vi "Step_Delay_Tommaso.vi"() -> ()   [LabVIEW 2015]
uses:
  <vilib>/DAQmx/write.llb/DAQmx Write (Analog DBL 1Chan 1Samp).vi
  <vilib>/DAQmx/miscellaneous.llb/DAQmx Fill In Error Info.vi
  <vilib>/DAQmx/create/channels.llb/DAQmx Create Channel (AO-Voltage-Basic).vi
  <vilib>/Analysis/1siggen.llb/Ramp Pattern by Delta.vi
  subvi/Newport ESP301/Newport ESP301.lvlib
  <vilib>/Analysis/NI_AALBase.lvlib
panel:
  in  "Dwell_positions":string[][](table)=[["-500", "3000"], ["-100", "3000"], ["0", "5000"], ["100", "5000"], ["500", "5000"], ["750", "10000"], ["1000", "10000"], ["", ""]]
  in  "Enable2":bool caption="Enable?"
  in  "Wait time [ms]":u32=1000 caption="Values <50 \nwon't work"
  out "StepSize [mm]":dbl=0.14989622900000002
  in  "stop 2":bool
  in  "StepSize [fs]":i32=1000
  in  "Enable?":bool
  out "a":waveform(dbl)(graph)={"t0"=timestamp(3629703941.150015 s since 1904-01-01), "dt"=1.0, "Y"=[-1.00695]}
  out "Waveform Chart":dbl(graph)=5.25341140860948
  out "x*y":dbl=0.9998993703837595
  in  "physical channels":tag="Dev3/ao1"
  out "DAC error":errorcluster
  out "ESP error":errorcluster
  out "run?":bool
  in  "set_vel":bool
  in  "velocity [fs/s]":dbl=333.564095198152
  in  "vel_mm":dbl=0.05 caption="velocity [mm/s]"
  out "meas. velocity":dbl
  in  "stop":bool
  out "output voltage":dbl=0.9998993703837595
  in  "start":bool
  in  "go2p1":bool
  out "position [mm]":dbl=-1.00695
  in  "p2 [mm]":dbl=-0.707153771
  in  "p1 [mm]":dbl=-1.006946229
  in  "interpolate output":bool
  in  "Delta2 [fs]":dbl=999.9999999999999
  in  "Delta1 [fs]":dbl=-999.9999999999999
  in  "Reference [mm]":dbl=-0.85705
  in  "Axis (1)":i32=3 min=1 max=3
  in  "Serial Link (RS232)":enum16{"RS232", "USB"}(ring)
  in  "VISA resource name":refnum<visa-resource-name>="COM9"
  in  "main_close":bool
  # "Interface panel"
  # "Velocity panel"
  # "Positions panel"
  # "Equally spaced steps panel"
  # "Controls panel"
  # "User-defined steps panel"
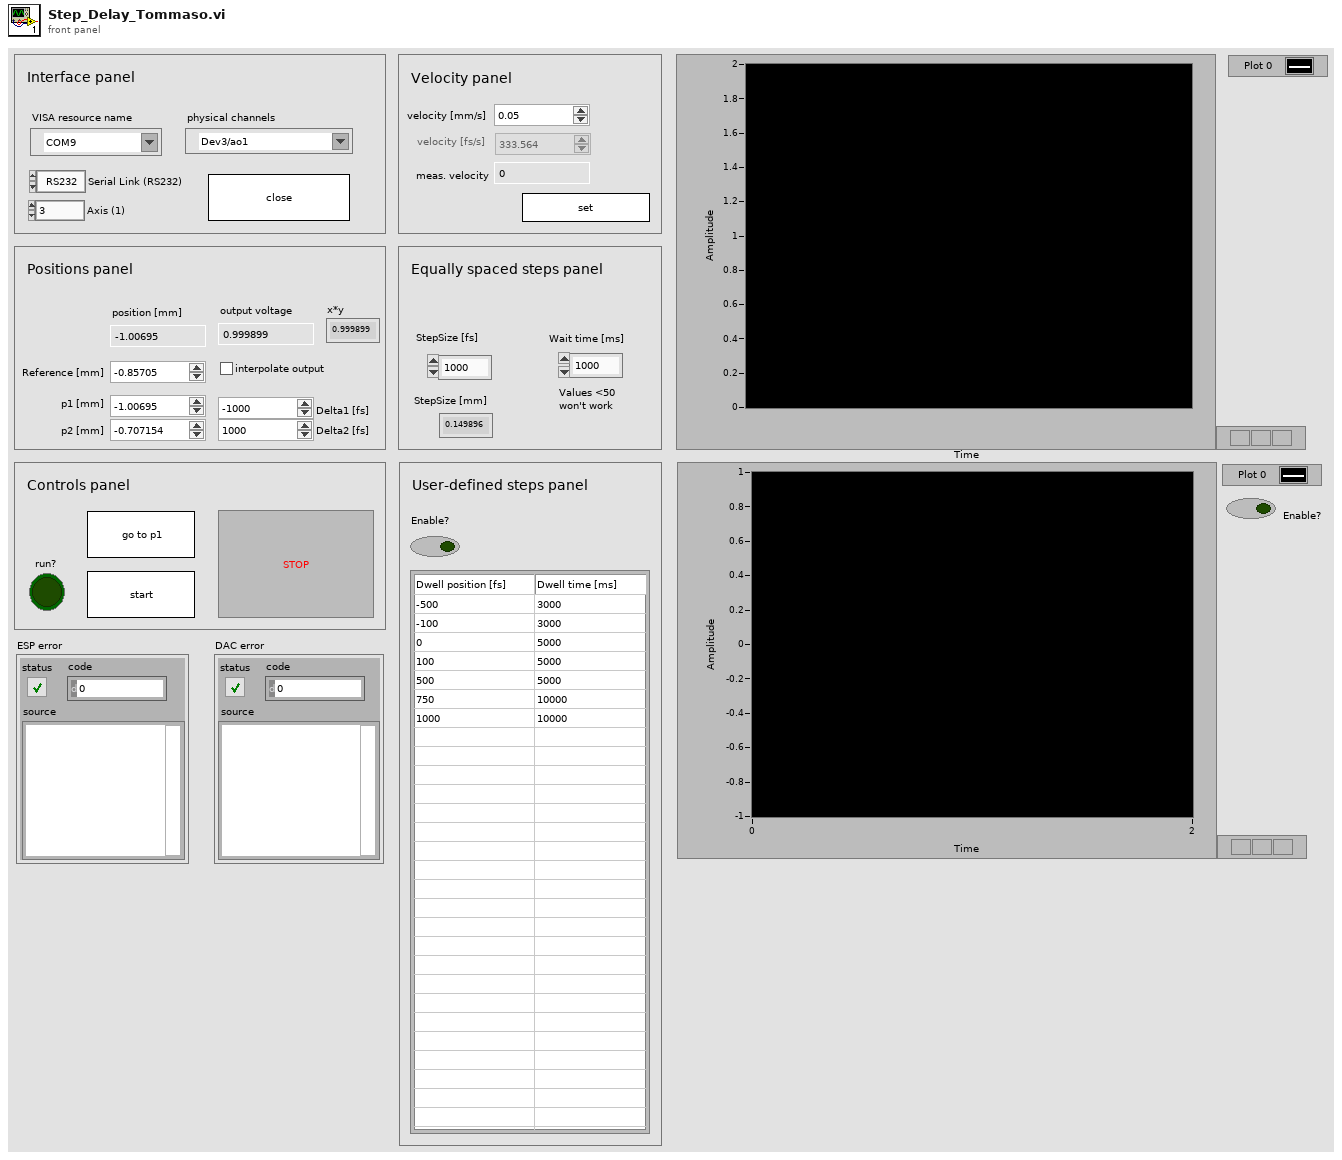
[diagram p1: front panel]
types:
  T1 = cluster{"dev1_data":refnum<queue>, "dev2_data":refnum<queue>}
  T2 = cluster{"dev1_cmd":refnum<queue>, "dev2_cmd":refnum<queue>}
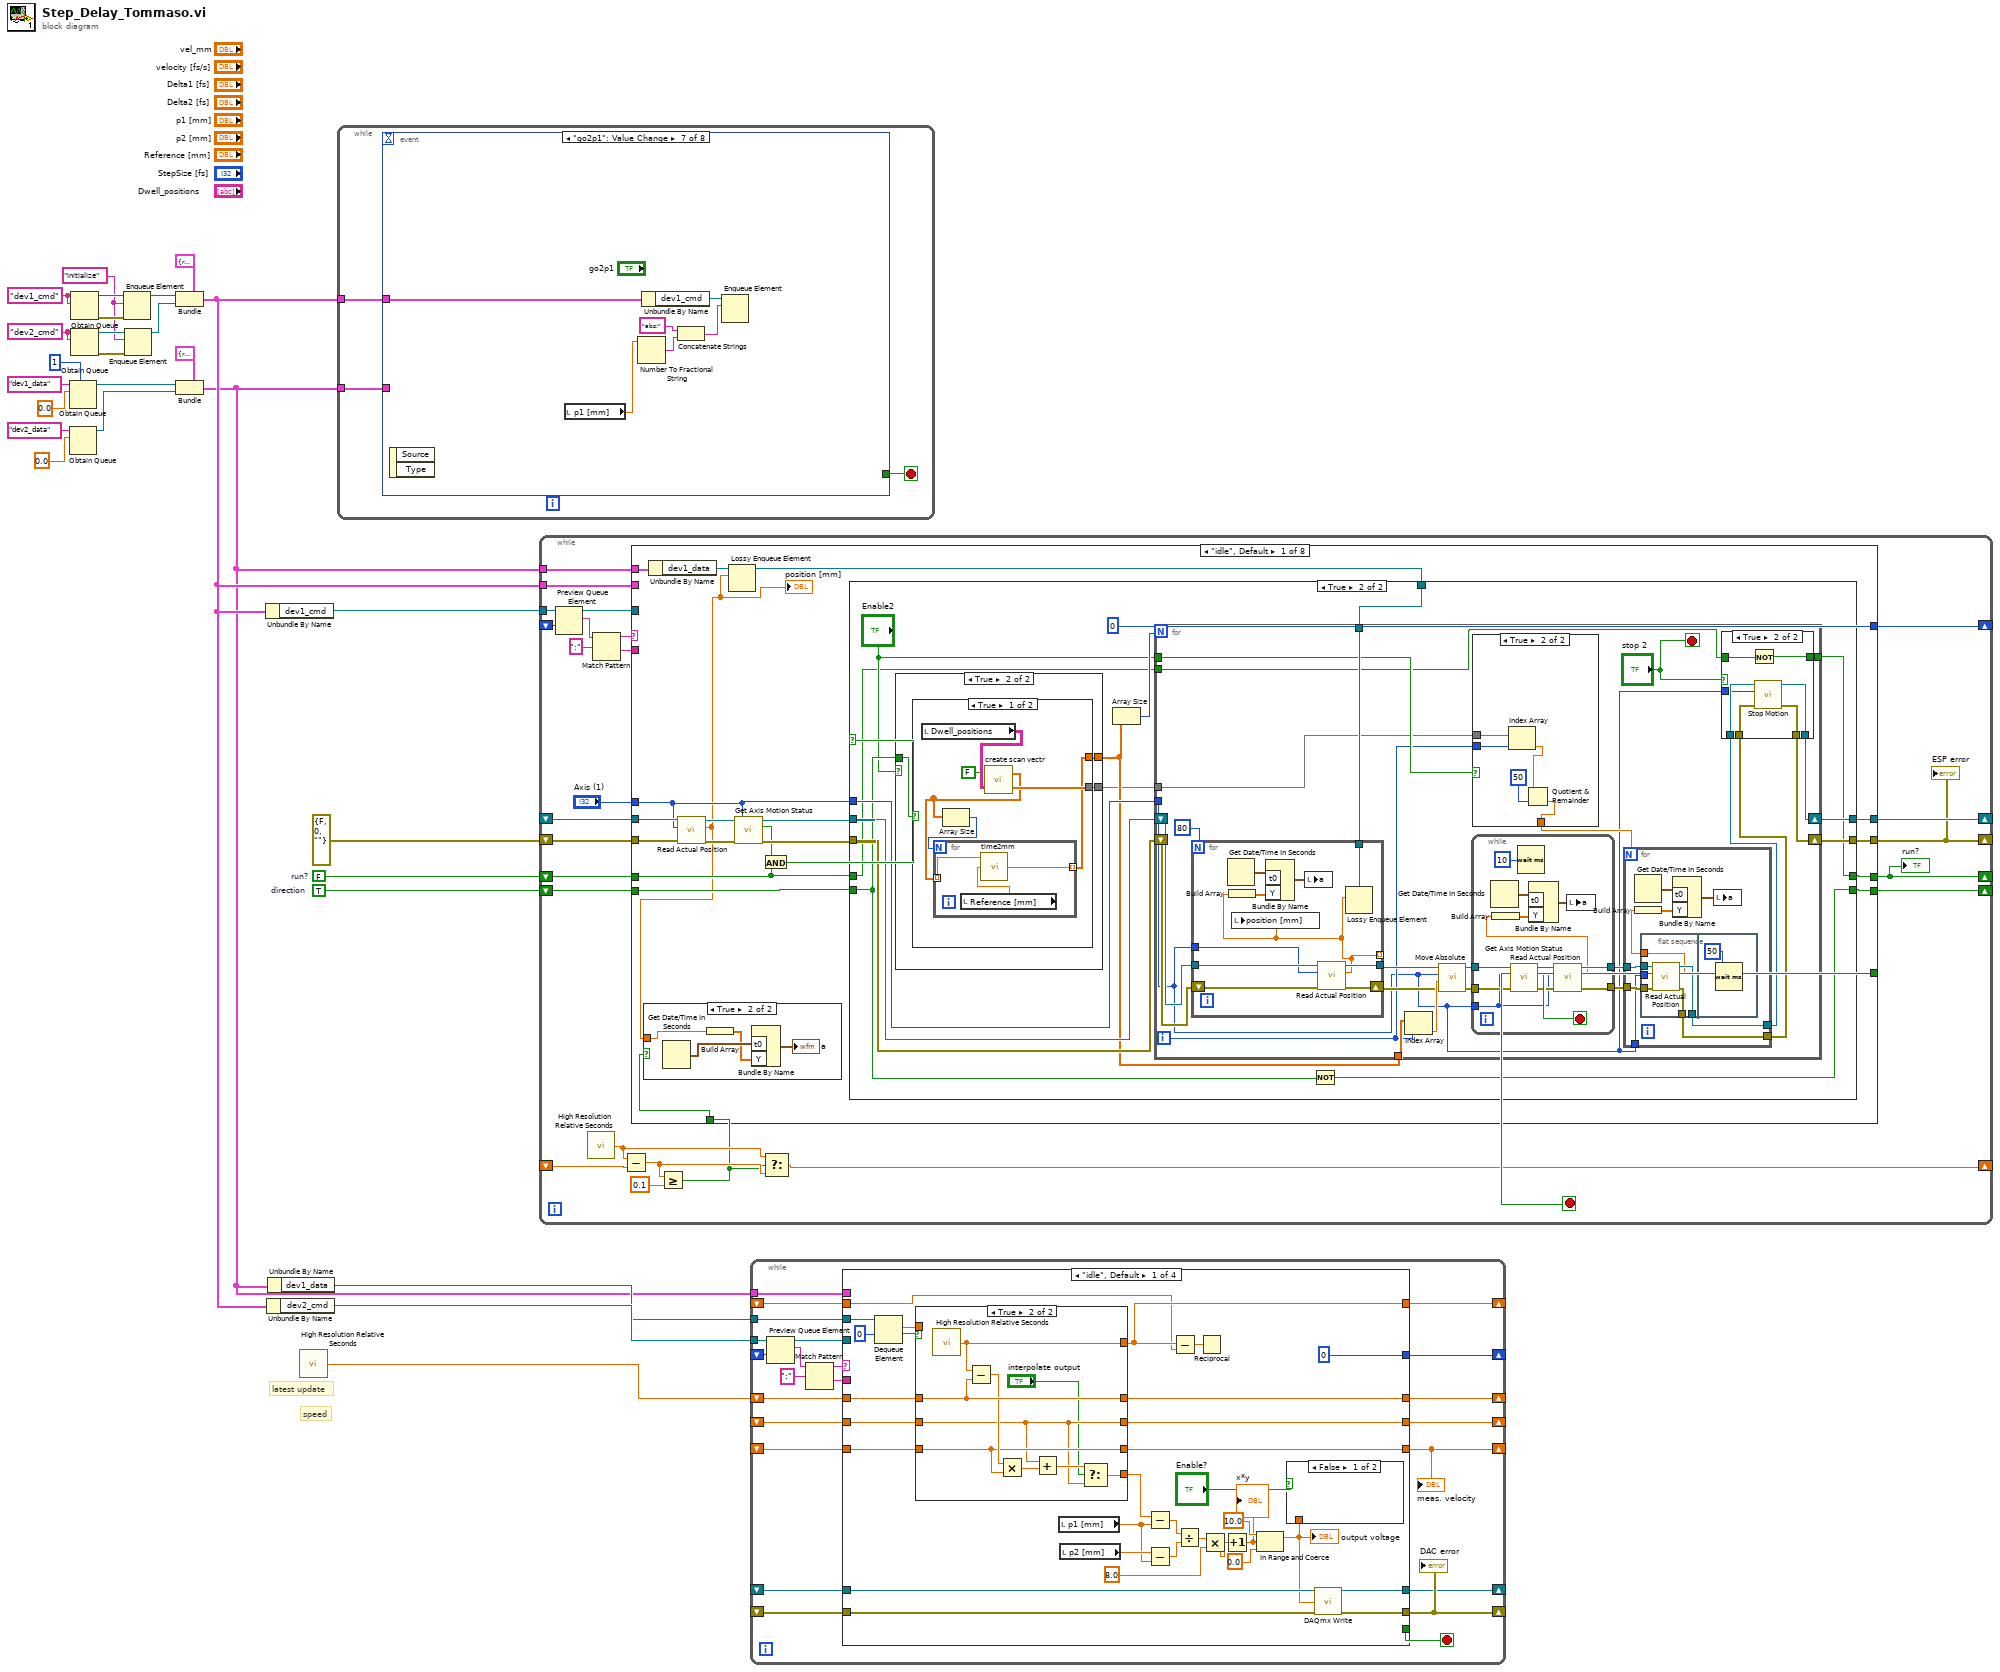
[diagram p0: block diagram]
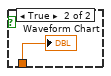
[diagram p2: hidden frame]
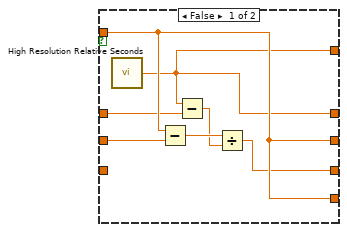
[diagram p3: hidden frame]
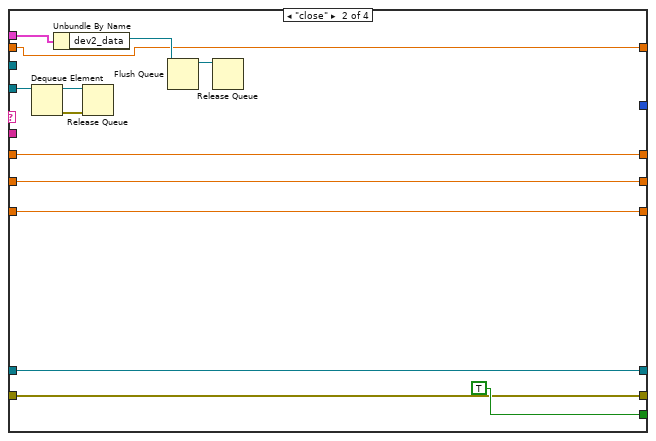
[diagram p4: hidden frame]
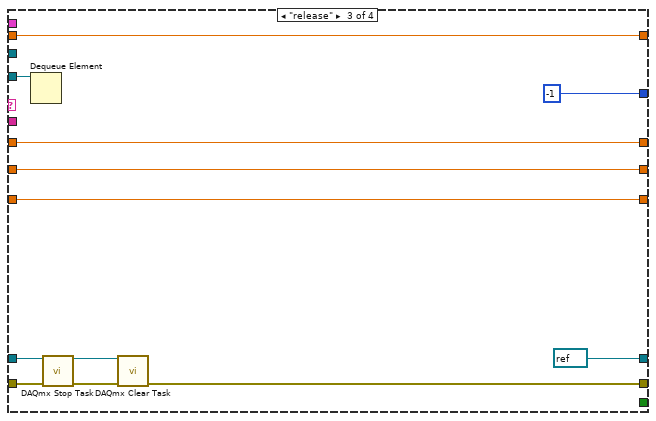
[diagram p5: hidden frame]
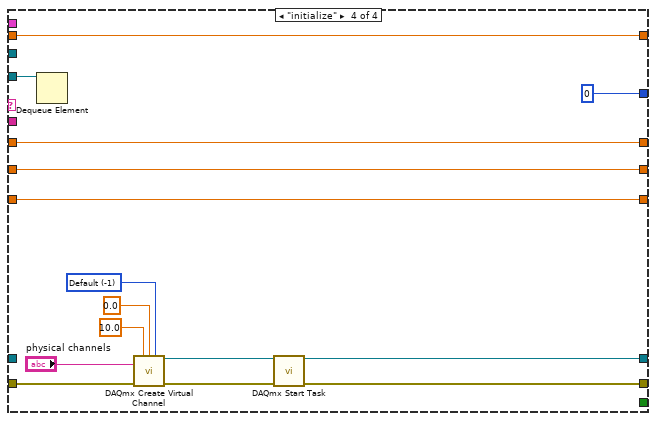
[diagram p6: hidden frame]
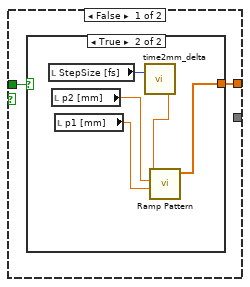
[diagram p9: hidden frame]
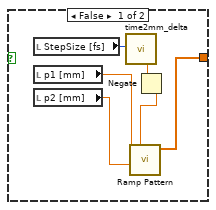
[diagram p10: hidden frame]
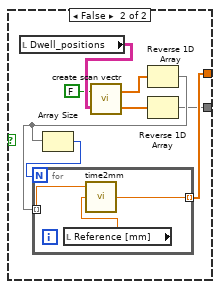
[diagram p11: hidden frame]
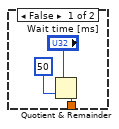
[diagram p13: hidden frame]
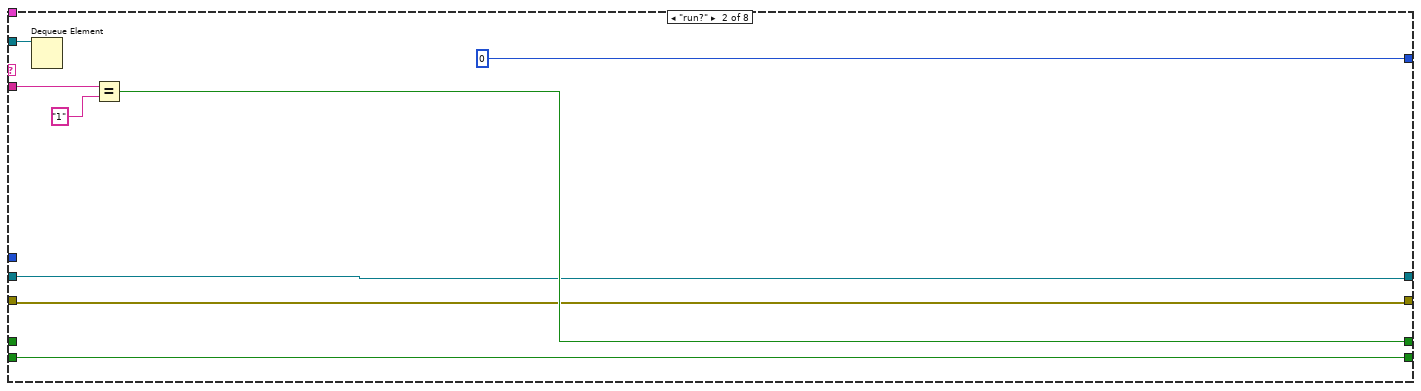
[diagram p14: hidden frame]
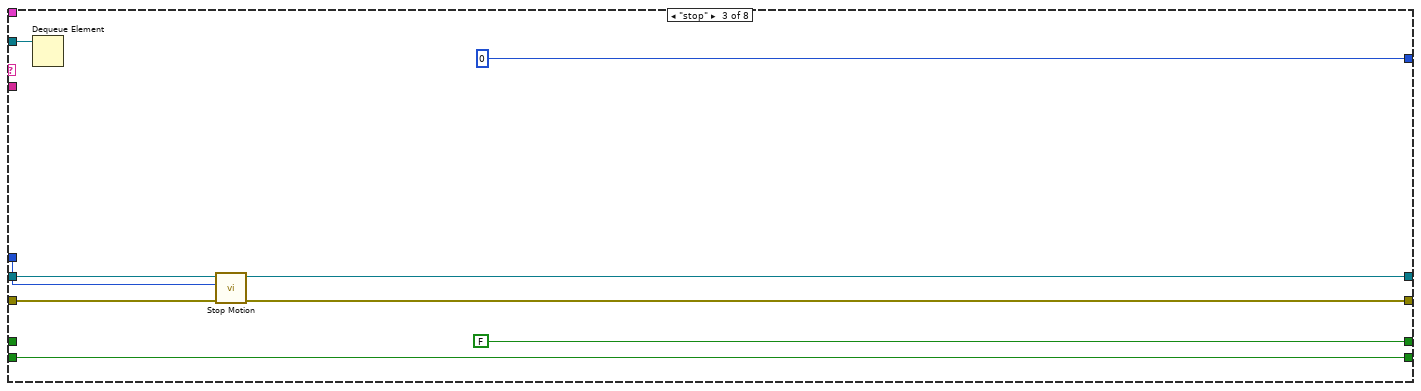
[diagram p15: hidden frame]
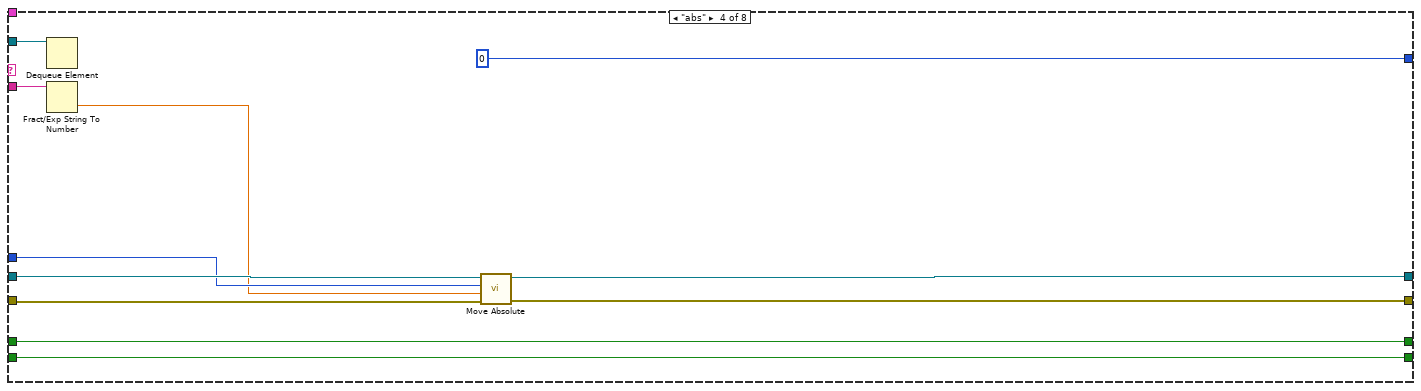
[diagram p16: hidden frame]
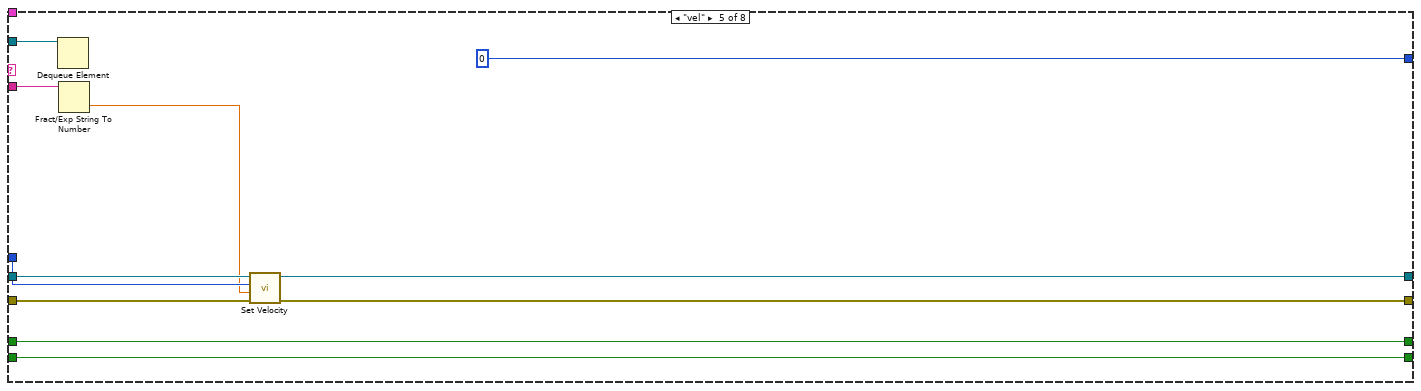
[diagram p17: hidden frame]
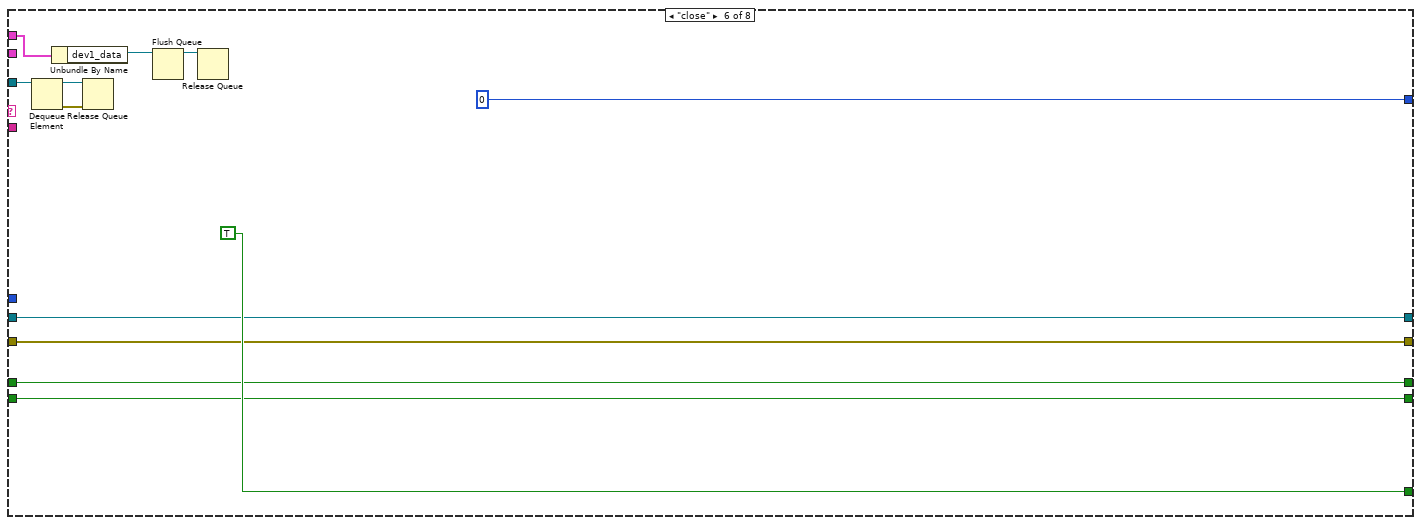
[diagram p18: hidden frame]
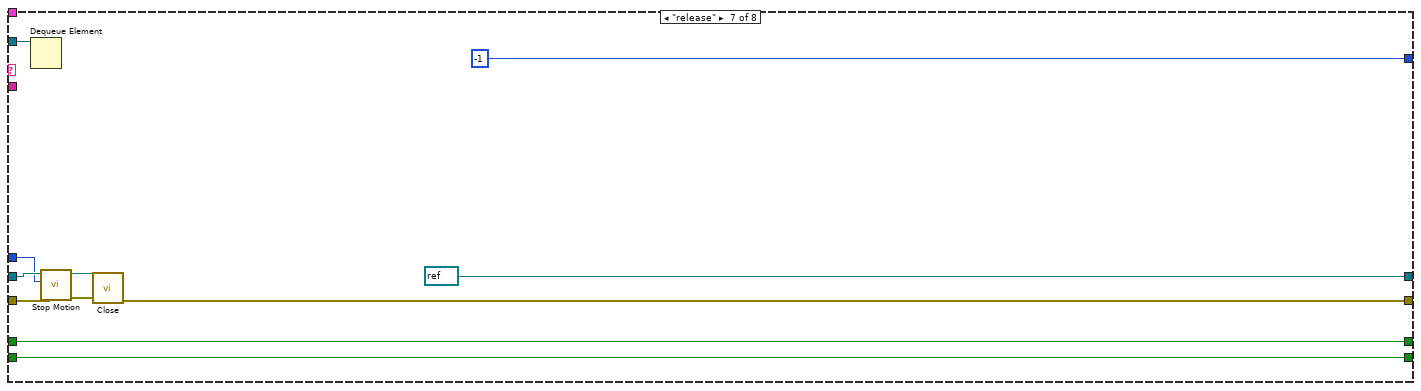
[diagram p19: hidden frame]
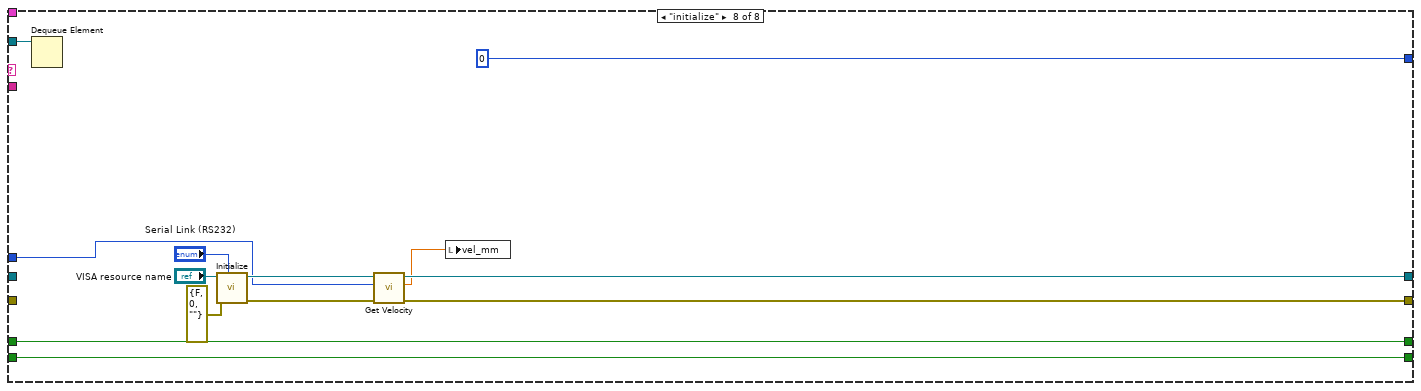
[diagram p20: hidden frame]
diagram:
  w1 = TRUE  # direction
  w4 = FALSE  # run?
  w15 = "dev2_cmd" ("name (unnamed)")
  w21 = "initialize" ("element")
  w16 = "dev1_cmd" ("name (unnamed)")
  # "speed"
  # "latest update"
  n1 = Obtain Queue(max queue size (-1, unlimited)=1, name (unnamed)="dev1_data", element data type=0.0) -> (queue out=w12:refnum<queue>)  [unwired: 2 in, 2 out]
  n2 = Obtain Queue(name (unnamed)="dev2_data", element data type=0.0) -> (queue out=w11:refnum<queue>)  [unwired: 3 in, 2 out]
  n3 = Obtain Queue(name (unnamed)=w16, element data type=w16) -> (queue out=w27:refnum<queue>, error out=w26:errorcluster)  [unwired: 3 in, 1 out]
  n4 = Obtain Queue(name (unnamed)=w15, element data type=w15) -> (queue out=w22:refnum<queue>, error out=w23:errorcluster)  [unwired: 3 in, 1 out]
  n5 = Enqueue Element(queue=w27, element=w21, error in (no error)=w26) -> (queue out=w24:refnum<queue>)  [unwired: 1 in, 2 out]
  n6 = Enqueue Element(queue=w22, element=w21, error in (no error)=w23) -> (queue out=w20:refnum<queue>)  [unwired: 1 in, 2 out]
  n7 = Bundle(cluster=T2 {"dev1_cmd"=refnum, "dev2_cmd"=refnum}, "dev1_cmd"=w24, "dev2_cmd"=w20) -> (w8:T2)
  n8 = Bundle(cluster=T1 {"dev1_data"=refnum, "dev2_data"=refnum}, "dev1_data"=w12, "dev2_data"=w11) -> (w2:T1)
  n9 = Unbundle By Name(w8) -> ("dev1_cmd"=w17:refnum<queue>)
  n10 = Unbundle By Name(w8) -> ("dev2_cmd"=w7:refnum<queue>)
  n11 = Unbundle By Name(w2) -> ("dev1_data"=w6:refnum<queue>)
  n12 = call <vilib>:"High Resolution Relative Seconds.vi"() -> ("relative seconds"=w5:dbl)
  n13 = while {
    tunnel: w8 -> [w30]
    tunnel: w2 -> [w29]
    stop <- w28 stop-if-true
    n14 = event shown="[6] \"go2p1\": Value Change" {
      selector: _ -> [_ _ _ _ _ _ _ _]
      dyn-events: _ -> [_ _ _ _ _ _ _ _]
      timeout: _ -> [_ _ _ _ _ _ _ _]
      tunnel: w30 -> [_ w34 _ _ w46 _ w64 w67]
      tunnel: w29 -> [_ _ _ _ _ _ _ _]
      tunnel: [_ _ _ _ _ _ _ TRUE] -> w28
      event Timeout {
        n15 = event-data() -> ()  [unwired: 1 in, 1 out]
      }
      event "start", "stop": Value Change {
        n16 = event-data() -> ()  [unwired: 1 in, 1 out]
        n17 = Boolean To (0,1)(Boolean="start") -> (0, 1=w32:i16)
        n18 = Number To Decimal String(number=w32) -> (decimal integer string=w31:string)  [unwired: 1 in]
        n19 = Unbundle By Name(w34) -> ("dev1_cmd"=w37:refnum<queue>)
        n20 = Concatenate Strings("run?:" ("string"), w31) -> (w36:string)
        n21 = Enqueue Element(queue=w37, element=w36) -> ()  [unwired: 2 in, 3 out]
      }
      event "StepSize [fs]": Value Change {
        n22 = event-data() -> ("NewVal"=w38:i32)  [unwired: 1 in, 5 out]
        n23 = call "time2mm_delta.vi"("Delta time"=w38) -> ("Delta position (mm)"=→"StepSize [mm]":dbl)  [unwired: 2 in]
      }
      event "Delta1 [fs]", "Delta2 [fs]": Value Change {
        n24 = event-data() -> ()  [unwired: 1 in, 1 out]
        n25 = local read "Reference [mm]"() -> (w41:dbl)
        n26 = local read "Delta2 [fs]"() -> (w42:dbl)
        n27 = local read "Delta1 [fs]"() -> (w44:dbl)
        n28 = call "time2mm.vi"("Offset (mm)"=w41, "time"=w44) -> ("position (mm)"=w43:dbl)  [unwired: 1 in]
        n29 = call "time2mm.vi"("Offset (mm)"=w41, "time"=w42) -> ("position (mm)"=w40:dbl)  [unwired: 1 in]
        n30 = local write "p2 [mm]"(w40) -> ()
        n31 = local write "p1 [mm]"(w43) -> ()
      }
      event "set_vel": Value Change {
        n32 = event-data() -> ()  [unwired: 1 in, 2 out]
        n33 = local read "vel_mm"() -> (w45:dbl)
        n34 = Number To Fractional String(number=w45) -> (F-format string=w49:string)  [unwired: 3 in]
        n35 = Unbundle By Name(w46) -> ("dev1_cmd"=w50:refnum<queue>)
        n36 = Concatenate Strings("vel:" ("string"), w49) -> (w48:string)
        n37 = Enqueue Element(queue=w50, element=w48) -> ()  [unwired: 2 in, 3 out]
      }
      event "p1 [mm]", "p2 [mm]", "Reference [mm]", "vel_mm": Value Change {
        n38 = event-data() -> ()  [unwired: 1 in, 2 out]
        n39 = local read "Reference [mm]"() -> (w56:dbl)
        n40 = local read "vel_mm"() -> (w53:dbl)
        n41 = local read "p1 [mm]"() -> (w57:dbl)
        n42 = local read "p2 [mm]"() -> (w58:dbl)
        n43 = call "mm2time.vi"("Offset (mm)"=0.0, "distance (mm)"=w53) -> ("time in fs"=w52:dbl)  [unwired: 1 in]
        n44 = call "mm2time.vi"("Offset (mm)"=w56, "distance (mm)"=w57) -> ("time in fs"=w54:dbl)  [unwired: 1 in]
        n45 = call "mm2time.vi"("Offset (mm)"=w56, "distance (mm)"=w58) -> ("time in fs"=w55:dbl)  [unwired: 1 in]
        n46 = local write "velocity [fs/s]"(w52) -> ()
        n47 = local write "Delta1 [fs]"(w54) -> ()
        n48 = local write "Delta2 [fs]"(w55) -> ()
      }
      event "go2p1": Value Change {
        n49 = event-data() -> ()  [unwired: 1 in, 2 out]
        n50 = local read "p1 [mm]"() -> (w59:dbl)
        n51 = Number To Fractional String(number=w59) -> (F-format string=w62:string)  [unwired: 3 in]
        n52 = Unbundle By Name(w64) -> ("dev1_cmd"=w63:refnum<queue>)
        n53 = Concatenate Strings("abs:" ("string"), w62) -> (w60:string)
        n54 = Enqueue Element(queue=w63, element=w60) -> ()  [unwired: 2 in, 3 out]
      }
      event "main_close": Value Change {
        n55 = event-data() -> ()  [unwired: 1 in, 1 out]
        n56 = Cluster To Array(cluster=w67) -> (array=w66:refnum<queue>[])
        n57 = for {
          tunnel: w66 -> [w72] mode=indexing
          n58 = Flush Queue(queue=w72) -> (queue out=w68:refnum<queue>)  [unwired: 1 in, 2 out]
          n59 = Enqueue Element(queue=w68, element="release") -> (queue out=w70:refnum<queue>)  [unwired: 2 in, 2 out]
          n60 = Enqueue Element(queue=w70, element="close") -> ()  [unwired: 2 in, 3 out]
        }
      }
    }
  }
  n61 = while {
    tunnel: w8 -> [w93]
    tunnel: w17 -> [w98]
    tunnel: w2 -> [w90]
    shift-right: [w88] -> _
    shift-left: _ -> [w89]
    shift-right: [w87] -> _
    shift-left: _ -> [w84]
    shift-right: [w86] -> _
    shift-left: errorcluster {"status"=FALSE, "code"=0, "source"=""} ("error out") -> [w85]
    shift-right: [w81] -> _
    shift-left: w4 -> [w82]
    shift-right: [w79] -> _
    shift-left: w1 -> [w80]
    shift-right: [w73] -> _
    shift-left: _ -> [w78]
    stop <- w91 stop-if-true
    n62 = Preview Queue Element(queue=w98, timeout in ms (-1)=w89) -> (queue out=w92:refnum<queue>, element=w97:string)  [unwired: 1 in, 2 out]
    n63 = call <vilib>:"High Resolution Relative Seconds.vi"() -> ("relative seconds"=w75:dbl)
    n64 = Match Pattern(string=w97, regular expression=":") -> (before substring=w95:string, after substring=w94:string)  [unwired: 1 in, 2 out]
    n65 = Subtract(x=w75, y=w78) -> (x-y=w76:dbl)
    n66 = Greater Or Equal?(x=w76, y=0.1) -> (x >= y?=w74:bool)
    n67 = case shown="\"idle\", Default" w95 {
      tunnel: w94 -> [_ w266 _ w285 w292 _ _ _]
      tunnel: w93 -> [_ _ _ _ _ _ _ _]
      tunnel: w92 -> [_ w264 w268 w286 w290 w309 w319 w329]
      tunnel: [_ _ _ _ _ TRUE _ _] -> w91
      tunnel: w90 -> [w118 _ _ _ _ w301 _ _]
      tunnel: [0 0 0 0 0 0 -1 0] -> w88
      tunnel: [w116 w259 w273 w282 w297 w305 refnum<visa-resource-name> refnum ("VISA resource name out") w325] -> w87
      tunnel: [w115 w260 w272 w281 w296 w304 w318 w324] -> w86
      tunnel: w85 -> [w113 w260 w274 w283 w295 w304 w314 _]
      tunnel: w84 -> [w114 w259 w275 w284 w294 w305 w311 _]
      tunnel: "Axis (1)" -> [w104 _ w271 w280 w293 _ w310 w326]
      tunnel: w82 -> [w102 _ _ w277 w288 w302 w316 w330]
      tunnel: [w110 w262 FALSE ("run?") w277 w288 w302 w316 w330] -> w81
      tunnel: w80 -> [w111 w261 w267 w276 w287 w298 w315 w321]
      tunnel: [w112 w261 w267 w276 w287 w298 w315 w321] -> w79
      tunnel: w74 -> [w99 _ _ _ _ _ _ _]
      frame "idle", Default {
        n68 = Unbundle By Name(w118) -> ("dev1_data"=w117:refnum<queue>)
        n69 = call "Read Actual Position.vi"("error in (no error)"=w113, "Axis (1)"=w104, "VISA resource name"=w114) -> ("error out"=w107:errorcluster, "Position (units)"=w100:dbl, "VISA resource name out"=w108:refnum<visa-resource-name>)  [unwired: 2 in]
        "position [mm]" <- w100
        n70 = case shown="True" w99 {
          tunnel: w100 -> [_ w123]
          frame False {
          }
          frame True {
            n71 = Get Date/Time In Seconds() -> (seconds since 1Jan1904=w122:timestamp)
            n72 = Build Array(w123) -> (w121:dbl[])
            n73 = Bundle By Name("t0"=w122, "Y"=w121) -> (→"a":waveform(dbl))  [unwired: 1 in]
          }
        }
        n74 = Lossy Enqueue Element(queue=w117, element=w100) -> (queue out=w109:refnum<queue>)  [unwired: 1 in, 3 out]
        n75 = call "Get Axis Motion Status.vi"("error in (no error)"=w107, "Axis (1)"=w104, "VISA resource name"=w108) -> ("error out"=w105:errorcluster, "Motion Done"=w103:bool, "VISA resource name out"=w106:refnum<visa-resource-name>)  [unwired: 2 in]
        n76 = And(x=w103, y=w102) -> (x .and. y?=w101:bool)
        n77 = case shown="True" w101 {
          tunnel: w106 -> [w127 w139]
          tunnel: w105 -> [w126 w140]
          tunnel: [w127 w138] -> w116
          tunnel: [w126 w137] -> w115
          tunnel: w104 -> [_ w136]
          tunnel: [w125 w135] -> w112
          tunnel: w111 -> [w125 w134]
          tunnel: w102 -> [w124 w129]
          tunnel: [w124 w128] -> w110
          tunnel: w109 -> [_ w141]
          frame False {
          }
          frame True {
            n78 = case shown="True" "Enable2" {
              tunnel: w134 -> [w143 w155]
              tunnel: [w142 w156] -> w133
              tunnel: [_ w157] -> w130
              frame False {
                n79 = case shown="True" w143 {
                  tunnel: [w147 w152] -> w142
                  frame False {
                    n80 = local read "StepSize [fs]"() -> (w144:i32)
                    n81 = local read "p1 [mm]"() -> (w149:dbl)
                    n82 = local read "p2 [mm]"() -> (w148:dbl)
                    n83 = call "time2mm_delta.vi"("Delta time"=w144) -> ("Delta position (mm)"=w145:dbl)  [unwired: 2 in]
                    n84 = Negate(x=w145) -> (-x=w146:dbl)
                    n85 = call-poly <vilib>:"Ramp Pattern.vi"("start"=w148, "end"=w149, "delta"=w146) -> ("Ramp Pattern"=w147:dbl[])  [unwired: 6 in, 2 out]
                  }
                  frame True {
                    n86 = local read "StepSize [fs]"() -> (w150:i32)
                    n87 = local read "p2 [mm]"() -> (w153:dbl)
                    n88 = local read "p1 [mm]"() -> (w154:dbl)
                    n89 = call "time2mm_delta.vi"("Delta time"=w150) -> ("Delta position (mm)"=w151:dbl)  [unwired: 2 in]
                    n90 = call-poly <vilib>:"Ramp Pattern.vi"("start"=w154, "end"=w153, "delta"=w151) -> ("Ramp Pattern"=w152:dbl[])  [unwired: 6 in, 2 out]
                  }
                }
              }
              frame True {
                n91 = case shown="True" w155 {
                  tunnel: [w161 w167] -> w157
                  tunnel: [w160 w172] -> w156
                  frame True {
                    n92 = local read "Dwell_positions"() -> (w163:string[][])
                    n93 = call "create scan vectr.vi"("Table Control"=w163, "waypoint mode?"=FALSE) -> ("Array 2"=w161:dbl[], "Array"=w159:dbl[])
                    n94 = Array Size(array=w159) -> (size(s)=w158:i32)
                    n95 = for {
                      N: w158 -> [_]
                      tunnel: w159 -> [w166] mode=indexing
                      tunnel: [w165] -> w160 mode=indexing
                      n96 = local read "Reference [mm]"() -> (w164:dbl)
                      n97 = call "time2mm.vi"("Offset (mm)"=w164, "time"=w166) -> ("position (mm)"=w165:dbl)  [unwired: 1 in]
                    }
                  }
                  frame False {
                    n98 = local read "Dwell_positions"() -> (w174:string[][])
                    n99 = call "create scan vectr.vi"("Table Control"=w174, "waypoint mode?"=FALSE) -> ("Array 2"=w168:dbl[], "Array"=w169:dbl[])
                    n100 = Reverse 1D Array(array=w169) -> (reversed array=w170:dbl[])
                    n101 = Array Size(array=w170) -> (size(s)=w171:i32)
                    n102 = for {
                      N: w171 -> [_]
                      tunnel: w170 -> [w177] mode=indexing
                      tunnel: [w176] -> w172 mode=indexing
                      n103 = local read "Reference [mm]"() -> (w175:dbl)
                      n104 = call "time2mm.vi"("Offset (mm)"=w175, "time"=w177) -> ("position (mm)"=w176:dbl)  [unwired: 1 in]
                    }
                    n105 = Reverse 1D Array(array=w168) -> (reversed array=w167:dbl[])
                  }
                }
              }
            }
            n106 = Array Size(array=w133) -> (size(s)=w132:i32)
            n107 = for {
              N: w132 -> [_]
              tunnel: w141 -> [w201]
              tunnel: w136 -> [w180]
              tunnel: w133 -> [w195]
              shift-right: [w182] -> w137
              shift-left: w140 -> [w199]
              shift-right: [w184] -> w138
              shift-left: w139 -> [w198]
              tunnel: "Enable2" -> [w188]
              tunnel: w130 -> [w186]
              tunnel: w129 -> [w179]
              tunnel: [w178] -> w128
              i -> [w187]
              stop <- "stop 2" stop-if-true
              n108 = for {
                N: 80 -> [_]
                tunnel: w198 -> [w258]
                tunnel: [w257] -> w197
                shift-right: [w253] -> w192
                shift-left: w199 -> [w256]
                tunnel: w180 -> [w255]
                tunnel: w201 -> [w254]
                tunnel: [w250] -> _ mode=indexing
                n109 = Get Date/Time In Seconds() -> (seconds since 1Jan1904=w251:timestamp)
                n110 = call "Read Actual Position.vi"("error in (no error)"=w256, "Axis (1)"=w255, "VISA resource name"=w258) -> ("error out"=w253:errorcluster, "Position (units)"=w250:dbl, "VISA resource name out"=w257:refnum<visa-resource-name>)  [unwired: 2 in]
                n111 = Build Array(w250) -> (w252:dbl[])
                n112 = local write "position [mm]"(w250) -> ()
                n113 = Bundle By Name("t0"=w251, "Y"=w252) -> (w249:waveform(dbl))  [unwired: 1 in]
                n114 = local write "a"(w249) -> ()
                n115 = Lossy Enqueue Element(queue=w254, element=w250) -> ()  [unwired: 1 in, 4 out]
              }
              n116 = Index Array(array=w195, index=w187) -> (element=w196:dbl)
              n117 = call "Move Absolute.vi"("error in (no error)"=w192, "Position (0 units)"=w196, "Axis (1)"=w180, "VISA resource name"=w197) -> ("error out"=w193:errorcluster, "VISA resource name out"=w194:refnum<visa-resource-name>)  [unwired: 2 in]
              n118 = while {
                tunnel: w194 -> [w248]
                tunnel: [w243] -> w189
                tunnel: w193 -> [w247]
                tunnel: [w241] -> w190
                tunnel: w180 -> [w240]
                stop <- w245 stop-if-true
                n119 = Get Date/Time In Seconds() -> (seconds since 1Jan1904=w239:timestamp)
                n120 = call "Get Axis Motion Status.vi"("error in (no error)"=w247, "Axis (1)"=w240, "VISA resource name"=w248) -> ("error out"=w242:errorcluster, "Motion Done"=w245:bool, "VISA resource name out"=w244:refnum<visa-resource-name>)  [unwired: 2 in]
                n121 = Wait (ms)(milliseconds to wait=10) -> ()  [unwired: 1 out]
                n122 = call "Read Actual Position.vi"("error in (no error)"=w242, "Axis (1)"=w240, "VISA resource name"=w244) -> ("error out"=w241:errorcluster, "Position (units)"=w237:dbl, "VISA resource name out"=w243:refnum<visa-resource-name>)  [unwired: 2 in]
                n123 = Build Array(w237) -> (w238:dbl[])
                n124 = Bundle By Name("t0"=w239, "Y"=w238) -> (w236:waveform(dbl))  [unwired: 1 in]
                n125 = local write "a"(w236) -> ()
              }
              n126 = case shown="True" w188 {
                tunnel: [w212 w218] -> w191
                tunnel: w187 -> [_ w216]
                tunnel: w186 -> [_ w215]
                frame False {
                  n127 = Quotient & Remainder(x="Wait time [ms]", y=50) -> (floor(x/y)=w212:u32)  [unwired: 1 out]
                }
                frame True {
                  n128 = Index Array(array=w215, index=w216) -> (element=w217:dbl)
                  n129 = Quotient & Remainder(x=w217, y=50) -> (floor(x/y)=w218:dbl)  [unwired: 1 out]
                }
              }
              n130 = for {
                N: w191 -> [_]
                tunnel: w190 -> [w228]
                tunnel: [w227] -> w183
                tunnel: w189 -> [w226]
                tunnel: [w225] -> w185
                tunnel: w180 -> [w224]
                n131 = Get Date/Time In Seconds() -> (seconds since 1Jan1904=w222:timestamp)
                n132 = Build Array(w221) -> (w223:dbl[])
                n133 = flat-sequence {
                  tunnel: w228 -> [w234]
                  tunnel: [w233] -> w227
                  tunnel: w226 -> [w232]
                  tunnel: [w231] -> w225
                  tunnel: w224 -> [w230]
                  tunnel: [w229] -> w221
                  frame #0 {
                    n134 = call "Read Actual Position.vi"("error in (no error)"=w234, "Axis (1)"=w230, "VISA resource name"=w232) -> ("error out"=w233:errorcluster, "Position (units)"=w229:dbl, "VISA resource name out"=w231:refnum<visa-resource-name>)  [unwired: 2 in]
                  }
                  frame #1 {
                    n135 = Wait (ms)(milliseconds to wait=50) -> ()  [unwired: 1 out]
                  }
                }
                n136 = Bundle By Name("t0"=w222, "Y"=w223) -> (w220:waveform(dbl))  [unwired: 1 in]
                n137 = local write "a"(w220) -> ()
              }
              n138 = case shown="True" "stop 2" {
                tunnel: w185 -> [w204 w211]
                tunnel: [w204 w210] -> w184
                tunnel: w183 -> [w203 w209]
                tunnel: [w203 w208] -> w182
                tunnel: w180 -> [_ w207]
                tunnel: w179 -> [w202 w206]
                tunnel: [w202 w205] -> w178
                frame False {
                }
                frame True {
                  n139 = Not(x=w206) -> (.not. x?=w205:bool)
                  n140 = call "Stop Motion.vi"("error in (no error)"=w209, "Axis (1)"=w207, "VISA resource name"=w211) -> ("error out"=w208:errorcluster, "VISA resource name out"=w210:refnum<visa-resource-name>)  [unwired: 3 in]
                }
              }
            }
            n141 = Not(x=w134) -> (.not. x?=w135:bool)
          }
        }
      }
      frame "run?" {
        n142 = Dequeue Element(queue=w264) -> ()  [unwired: 2 in, 4 out]
        n143 = Equal?(x=w266, y="1") -> (x = y?=w262:bool)
      }
      frame "stop" {
        n144 = Dequeue Element(queue=w268) -> ()  [unwired: 2 in, 4 out]
        n145 = call "Stop Motion.vi"("error in (no error)"=w274, "Axis (1)"=w271, "VISA resource name"=w275) -> ("error out"=w272:errorcluster, "VISA resource name out"=w273:refnum<visa-resource-name>)  [unwired: 3 in]
      }
      frame "abs" {
        n146 = Dequeue Element(queue=w286) -> ()  [unwired: 2 in, 4 out]
        n147 = Fract/Exp String To Number(string=w285) -> (number=w279:dbl)  [unwired: 3 in, 1 out]
        n148 = call "Move Absolute.vi"("error in (no error)"=w283, "Position (0 units)"=w279, "Axis (1)"=w280, "VISA resource name"=w284) -> ("error out"=w281:errorcluster, "VISA resource name out"=w282:refnum<visa-resource-name>)  [unwired: 2 in]
      }
      frame "vel" {
        n149 = Dequeue Element(queue=w290) -> ()  [unwired: 2 in, 4 out]
        n150 = Fract/Exp String To Number(string=w292) -> (number=w291:dbl)  [unwired: 3 in, 1 out]
        n151 = call "Set Velocity.vi"("error in (no error)"=w295, "Velocity (units/s)"=w291, "Axis (1)"=w293, "VISA resource name"=w294) -> ("error out"=w296:errorcluster, "VISA resource name out"=w297:refnum<visa-resource-name>)  [unwired: 2 in]
      }
      frame "close" {
        n152 = Dequeue Element(queue=w309) -> (queue out=w308:refnum<queue>, error out=w307:errorcluster)  [unwired: 2 in, 2 out]
        n153 = Unbundle By Name(w301) -> ("dev1_data"=w299:refnum<queue>)
        n154 = Release Queue(queue=w308, error in (no error)=w307) -> ()  [unwired: 1 in, 3 out]
        n155 = Flush Queue(queue=w299) -> (queue out=w300:refnum<queue>)  [unwired: 1 in, 2 out]
        n156 = Release Queue(queue=w300) -> ()  [unwired: 2 in, 3 out]
      }
      frame "release" {
        n157 = Dequeue Element(queue=w319) -> ()  [unwired: 2 in, 4 out]
        n158 = call "Stop Motion.vi"("error in (no error)"=w314, "Axis (1)"=w310, "VISA resource name"=w311) -> ("error out"=w313:errorcluster, "VISA resource name out"=w312:refnum<visa-resource-name>)  [unwired: 3 in]
        n159 = call "Close.vi"("error in (no error)"=w313, "VISA resource name"=w312) -> ("error out"=w318:errorcluster)  [unwired: 9 in]
      }
      frame "initialize" {
        n160 = Dequeue Element(queue=w329) -> ()  [unwired: 2 in, 4 out]
        n161 = call "Initialize.vi"("VISA resource name"="VISA resource name", "error in (no error)"=errorcluster {"status"=FALSE, "code"=0, "source"=""}, "Serial Link (RS232)"="Serial Link (RS232)") -> ("VISA resource name out"=w328:refnum<visa-resource-name>, "error out"=w327:errorcluster)  [unwired: 6 in]
        n162 = call "Get Velocity.vi"("error in (no error)"=w327, "Axis (1)"=w326, "VISA resource name"=w328) -> ("error out"=w324:errorcluster, "Velocity (units/s)"=w323:dbl, "VISA resource name out"=w325:refnum<visa-resource-name>)  [unwired: 2 in]
        n163 = local write "vel_mm"(w323) -> ()
      }
    }
    "run?" <- w81
    "ESP error" <- w86
    n164 = Select(t=w75, s=w74, f=w76) -> (s? t:f=w73:dbl)
  }
  n165 = while {
    shift-right: [w349] -> _
    shift-left: _ -> [w350]
    shift-right: [w348] -> _
    shift-left: _ -> [w347]
    tunnel: w7 -> [w346]
    shift-right: [w345] -> _
    shift-left: _ -> [w344]
    tunnel: w6 -> [w343]
    shift-right: [w342] -> _
    shift-left: _ -> [w339]
    shift-right: [w341] -> _
    shift-left: w5 -> [w340]
    shift-right: [w334] -> _
    shift-left: _ -> [w338]
    tunnel: w2 -> [w337]
    shift-right: [w336] -> _
    shift-left: _ -> [w335]
    stop <- w351 stop-if-true
    n166 = Preview Queue Element(queue=w346, timeout in ms (-1)=w350) -> (queue out=w352:refnum<queue>, element=w356:string)  [unwired: 1 in, 2 out]
    n167 = Match Pattern(string=w356, regular expression=":") -> (before substring=w354:string, after substring=w353:string)  [unwired: 1 in, 2 out]
    n168 = case shown="\"idle\", Default" w354 {
      tunnel: w353 -> [_ _ _ _]
      tunnel: w352 -> [_ w417 w428 w436]
      tunnel: [_ TRUE _ _] -> w351
      tunnel: [0 _ -1 0] -> w349
      tunnel: [w383 w413 w427 w437] -> w348
      tunnel: w347 -> [w381 w413 w424 w444]
      tunnel: [w384 w412 refnum<k21> refnum ("task out") w438] -> w345
      tunnel: w344 -> [w382 w412 w425 _]
      tunnel: w343 -> [w385 _ _ _]
      tunnel: [w379 w410 w420 w433] -> w342
      tunnel: [w378 w411 w421 w434] -> w341
      tunnel: w340 -> [w376 w411 w421 w434]
      tunnel: w339 -> [w377 w410 w420 w433]
      tunnel: [w375 w409 w419 w432] -> w334
      tunnel: w338 -> [w374 w409 w419 w432]
      tunnel: w337 -> [_ w406 _ _]
      tunnel: [w363 w405 w418 w430] -> w336
      tunnel: w335 -> [w362 w405 w418 w430]
      frame "idle", Default {
        n169 = Dequeue Element(queue=w385, timeout in ms (-1)=0) -> (element=w380:dbl, timed out?=w364:bool)  [unwired: 1 in, 2 out]
        n170 = case shown="True" w364 {
          tunnel: w380 -> [w395 _]
          tunnel: [w395 w397] -> w373
          tunnel: [w395 w399] -> w379
          tunnel: [w389 w404] -> w378
          tunnel: w377 -> [w394 w399]
          tunnel: w376 -> [w393 w404]
          tunnel: [w390 w401] -> w375
          tunnel: w374 -> [_ w401]
          tunnel: [w389 w396] -> w363
          frame False {
            n171 = call <vilib>:"High Resolution Relative Seconds.vi"() -> ("relative seconds"=w389:dbl)
            n172 = Subtract(x=w395, y=w394) -> (x-y=w392:dbl)
            n173 = Subtract(x=w389, y=w393) -> (x-y=w391:dbl)
            n174 = Divide(x=w392, y=w391) -> (x/y=w390:dbl)
          }
          frame True {
            n175 = call <vilib>:"High Resolution Relative Seconds.vi"() -> ("relative seconds"=w396:dbl)
            n176 = Subtract(x=w396, y=w404) -> (x-y=w403:dbl)
            n177 = Multiply(x=w403, y=w401) -> (x*y=w402:dbl)
            n178 = Add(x=w399, y=w402) -> (x+y=w400:dbl)
            n179 = Select(t=w400, s="interpolate output", f=w399) -> (s? t:f=w397:dbl)
          }
        }
        n180 = local read "p1 [mm]"() -> (w371:dbl)
        n181 = local read "p2 [mm]"() -> (w372:dbl)
        n182 = Subtract(x=w373, y=w371) -> (x-y=w370:dbl)
        n183 = Subtract(x=w372, y=w371) -> (x-y=w369:dbl)
        n184 = Subtract(x=w363, y=w362) -> (x-y=w361:dbl)
        n185 = Divide(x=w370, y=w369) -> (x/y=w368:dbl)
        n186 = Reciprocal(x=w361) -> ()  [unwired: 1 out]
        n187 = Multiply(x=w368, y=8.0) -> (x*y=w359:dbl)
        n188 = Increment(x=w359) -> (x+1=w358:dbl)
        "x*y" <- w358
        n189 = In Range and Coerce(upper limit=10.0, x=w358, lower limit=0.0) -> (coerced(x)=w360:dbl)  [unwired: 1 out]
        "output voltage" <- w360
        n190 = case shown="False" "Enable?" {
          tunnel: w360 -> [_ w388]
          frame False {
          }
          frame True {
            "Waveform Chart" <- w388
          }
        }
        n191 = call-poly <vilib>:"DAQmx Write.vi"("task/channels in"=w382, "data"=w360, "error in"=w381) -> ("task out"=w384:refnum<k21>, "error out"=w383:errorcluster)  [unwired: 10 in, 1 out]
      }
      frame "close" {
        n192 = Dequeue Element(queue=w417) -> (queue out=w416:refnum<queue>, error out=w415:errorcluster)  [unwired: 2 in, 2 out]
        n193 = Unbundle By Name(w406) -> ("dev2_data"=w407:refnum<queue>)
        n194 = Release Queue(queue=w416, error in (no error)=w415) -> ()  [unwired: 1 in, 3 out]
        n195 = Flush Queue(queue=w407) -> (queue out=w408:refnum<queue>)  [unwired: 1 in, 2 out]
        n196 = Release Queue(queue=w408) -> ()  [unwired: 2 in, 3 out]
      }
      frame "release" {
        n197 = Dequeue Element(queue=w428) -> ()  [unwired: 2 in, 4 out]
        n198 = call <vilib>:"DAQmx Stop Task.vi"("task/channels in"=w425, "error in"=w424) -> ("task out"=w423:refnum<k21>, "error out"=w422:errorcluster)  [unwired: 12 in]
        n199 = call <vilib>:"DAQmx Clear Task.vi"("task in"=w423, "error in"=w422) -> ("error out"=w427:errorcluster)  [unwired: 13 in]
      }
      frame "initialize" {
        w441 = -1 items=["Default"=-1, "RSE"=10083, "Differential"=10106, "Pseudodifferential"=12529] ("output terminal configuration")
        n200 = Dequeue Element(queue=w436) -> ()  [unwired: 2 in, 4 out]
        n201 = call-poly <vilib>:"DAQmx Create Virtual Channel.vi"("maximum value"=10.0, "minimum value"=0.0, "output terminal configuration"=w441, "physical channels"="physical channels", "error in"=w444) -> ("task out"=w440:refnum<k21>, "error out"=w439:errorcluster)  [unwired: 9 in]
        n202 = call <vilib>:"DAQmx Start Task.vi"("task/channels in"=w440, "error in"=w439) -> ("task out"=w438:refnum<k21>, "error out"=w437:errorcluster)  [unwired: 12 in]
      }
    }
    "meas. velocity" <- w334
    "DAC error" <- w348
  }
